vi "Get coordinates of visible image part.vi"(11 "Image Control":refnum<vi>) -> (2 "Bottom-right pixel":cluster{"x":i32, "y":i32}, 3 "Top-left pixel":cluster{"x":i32, "y":i32})   [LabVIEW 2011, in "COSYLib.lvlib"]
doc: "Returns the pixel coordinates (in the image's coordinate system) of the top-left and bottom-right pixels displayed in an <B>Image Control</B>.\n\nIf the full image is visible, the outermost pixel coordinates are returned. Otherwise, if the image doesn't fit in the viewport (because, for example, it is zoomed in), the top-left and bottom-right pixel coordinates are calculated.\n\nNote: the calculated coordinates might be one off; an exact calculation doesn't seem possible with the information available in an Image Display's property node."
uses:
  COSYLib.lvlib
  <vilib>/vision/Image Controls.llb/IMAQ Image.ctl
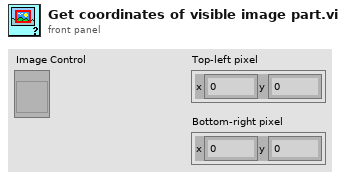
[diagram p1: front panel]
types:
  T1 = typedef "IMAQ Image.ctl" = refnum<image>
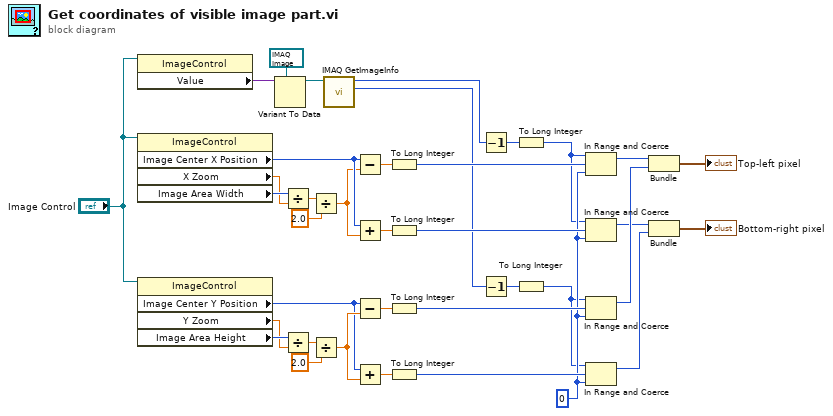
[diagram p0: block diagram]
diagram:
  w17 = 0 ("lower limit")
  n1 = property class="ImageControl"(reference="Image Control") -> ("Value"=w5:variant)  [unwired: 1 in, 2 out]
  n2 = property class="ImageControl"(reference="Image Control") -> ("Image Center X Position"=w33:u32, "X Zoom"=w36:sgl, "Image Area Width"=w37:u32)  [unwired: 1 in, 2 out]
  n3 = property class="ImageControl"(reference="Image Control") -> ("Image Center Y Position"=w28:u32, "Y Zoom"=w26:sgl, "Image Area Height"=w27:u32)  [unwired: 1 in, 2 out]
  n4 = Variant To Data(type=T1 refnum ("Image"), Variant=w5) -> (data=w3:T1)  [unwired: 1 in, 1 out]
  n5 = Divide(x=w37, y=w36) -> (x/y=w35:sgl)
  n6 = Divide(x=w27, y=w26) -> (x/y=w29:sgl)
  n7 = Divide(x=w35, y=sgl 2.0) -> (x/y=w32:sgl)
  n8 = Divide(x=w29, y=sgl 2.0) -> (x/y=w31:sgl)
  n9 = call "IMAQ GetImageInfo"("Image"=w3) -> ("Y Resolution"=w1:i32, "X Resolution"=w2:i32)  [unwired: 3 in, 6 out]
  n10 = Subtract(x=w33, y=w32) -> (x-y=w25:sgl)
  n11 = Add(x=w33, y=w32) -> (x+y=w24:sgl)
  n12 = Subtract(x=w28, y=w31) -> (x-y=w23:sgl)
  n13 = Add(x=w28, y=w31) -> (x+y=w22:sgl)
  n14 = To Long Integer(number=w25) -> (32bit integer=w21:i32)
  n15 = To Long Integer(number=w24) -> (32bit integer=w20:i32)
  n16 = To Long Integer(number=w23) -> (32bit integer=w19:i32)
  n17 = To Long Integer(number=w22) -> (32bit integer=w18:i32)
  n18 = Decrement(x=w2) -> (x-1=w16:i32)
  n19 = Decrement(x=w1) -> (x-1=w15:i32)
  n20 = To Long Integer(number=w16) -> (32bit integer=w13:i32)
  n21 = To Long Integer(number=w15) -> (32bit integer=w12:i32)
  n22 = In Range and Coerce(upper limit=w13, x=w21, lower limit=w17) -> (coerced(x)=w14:i32)  [unwired: 1 out]
  n23 = In Range and Coerce(upper limit=w13, x=w20, lower limit=w17) -> (coerced(x)=w10:i32)  [unwired: 1 out]
  n24 = In Range and Coerce(upper limit=w12, x=w19, lower limit=w17) -> (coerced(x)=w11:i32)  [unwired: 1 out]
  n25 = In Range and Coerce(upper limit=w12, x=w18, lower limit=w17) -> (coerced(x)=w9:i32)  [unwired: 1 out]
  n26 = Bundle("lower limit"=w14, "lower limit"=w11) -> (→"Top-left pixel":cluster{"lower limit":i32, "lower limit":i32})  [unwired: 1 in]
  n27 = Bundle("lower limit"=w10, "lower limit"=w9) -> (→"Bottom-right pixel":cluster{"lower limit":i32, "lower limit":i32})  [unwired: 1 in]
